vi "Start Game.vi"(10 "Board Size":i32, 11 "Team in":refnum<class "Team.lvclass">) -> (3 "Team out":refnum<class "Team.lvclass">)   [LabVIEW 2020, in "SquareBattle.lvlib" / "Team.lvclass"]
doc: "Called once at the start of every game before the first square is placed. This is an opportunity to create any shared resources needed during a game although sticking to dataflow and by-value mechanisms is highly encouraged. The team gets passed into every square call and its data maintained so there is no need for by-reference mechanisms as long as shared state is kept within the team class data."
uses:
  Team.lvclass
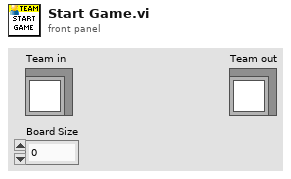
[diagram p1: front panel]
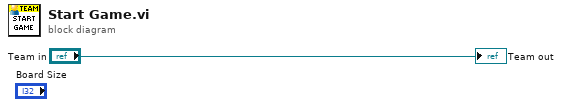
[diagram p0: block diagram]
diagram:
  "Team out" <- "Team in"
